vi "MinNode.vi"(9 "index":i32=1, 11 "Tree":dbl[][](array[numeric])) -> (1 "Min Node":dbl[](array[numeric]))   [LabVIEW 2016]
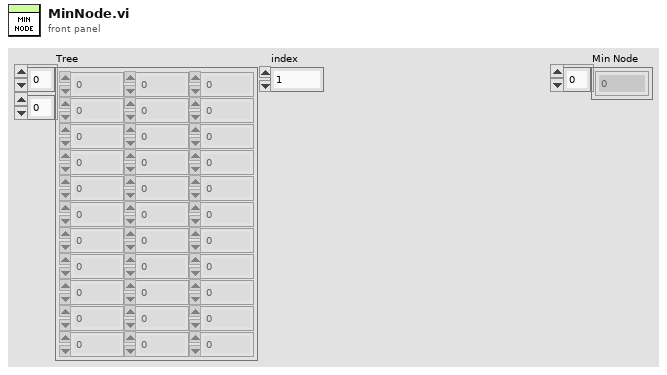
[diagram p1: front panel]
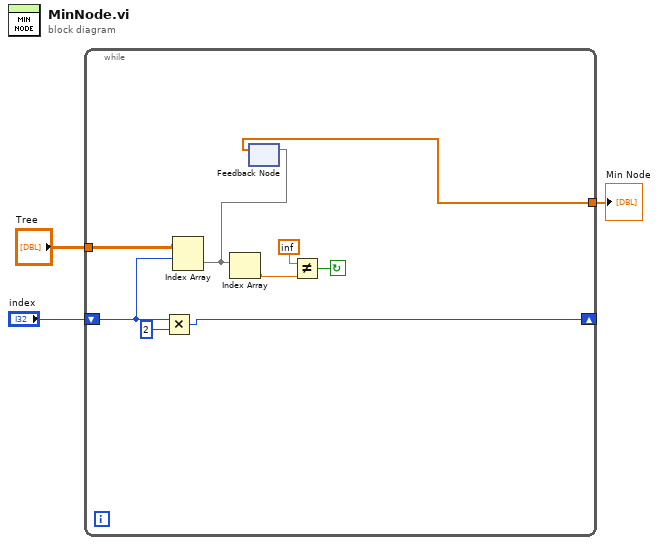
[diagram p0: block diagram]
diagram:
  n1 = while {
    tunnel: "Tree" -> [w12]
    shift-right: [w6] -> _
    shift-left: "index" -> [w8]
    tunnel: [w4] -> w1
    stop <- w9 continue-if-true
    n2 = Multiply(x=w8, y=2) -> (x*y=w6:i32)
    n3 = Index Array(array=w12, index (row)=w8) -> (element=w5:dbl[])  [unwired: 1 in]
    n4 = Index Array(array=w5) -> (element=w10:dbl)  [unwired: 1 in]
    n5 = feedback-in #1(w5) -> ()
    n6 = feedback #1() -> (w4:dbl[])  [unwired: 1 in]
    n7 = Not Equal?(x=inf, y=w10) -> (x != y?=w9:bool)
  }
  "Min Node" <- w1
